vi "add plugin to configuration.vi"(8 "error in (no error)":errorcluster, 9 "plugin info":T1, 10 "id":string, 11 "DSFConfiguration in":refnum<class "DSFConfiguration.lvclass">) -> (0 "error out":errorcluster, 3 "DSFConfiguration out":refnum<class "DSFConfiguration.lvclass">)   [LabVIEW 2017, in "DSFConfiguration.lvclass"]
uses:
  DSFConfiguration.lvclass
  Controls/dsf plugin.ctl
  Controls/dsf timing.ctl
  DSFConfiguration.lvclass/DSFConfiguration.ctl
  DSFPlugin/DSFPlugin.lvclass
  C:/github/data-sharing-framework/Source/Configuration API/Classes/IDable/IDable.lvclass
  IDable/IDable.lvclass/IDable.ctl
  ID API/ID API.lvclass
  IDable/IDable.lvclass
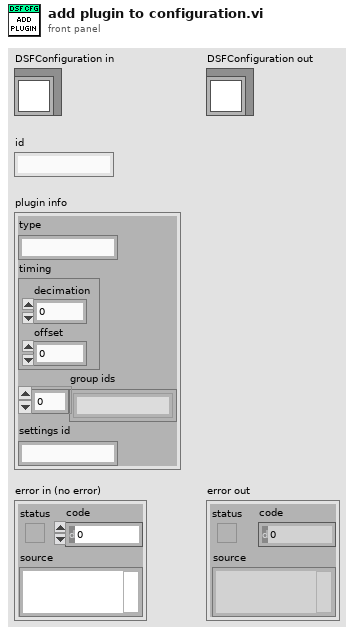
[diagram p1: front panel]
types:
  T1 = typedef "dsf plugin.ctl" = cluster{"type":string, "timing":T2, "group ids":string[], "settings id":string}
  T2 = typedef "dsf timing.ctl" = cluster{"decimation":i32, "offset":i32}
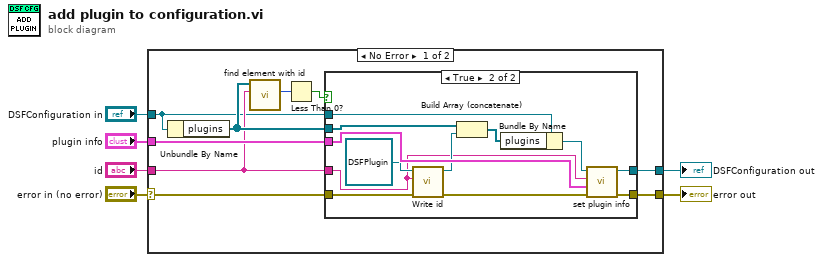
[diagram p0: block diagram]
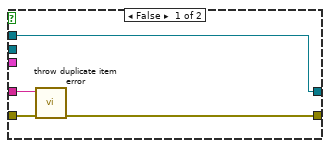
[diagram p2: hidden frame]
diagram:
  n1 = case shown="No Error" "error in (no error)" {
    selector: "error in (no error)" -> [w11 w33]
    tunnel: [w12 w33] -> w1
    tunnel: "DSFConfiguration in" -> [w7 w32]
    tunnel: "id" -> [w9 _]
    tunnel: "plugin info" -> [w10 _]
    tunnel: [w8 w32] -> w2
    frame No Error {
      n2 = Unbundle By Name(w7) -> ("plugins"=w13:refnum<class "DSFPlugin.lvclass">[])
      n3 = call "find element with id.vi"("id"=w9, "IDable Array in"=w13) -> ("index"=w15:i32)  [unwired: 8 in, 1 out]
      n4 = Less Than 0?(x=w15) -> (x < 0?=w14:bool)
      n5 = case shown="True" w14 {
        tunnel: w13 -> [_ w31]
        tunnel: [w19 w26] -> w12
        tunnel: w11 -> [w16 w30]
        tunnel: w10 -> [_ w24]
        tunnel: w9 -> [w17 w20]
        tunnel: w7 -> [w18 w29]
        tunnel: [w18 w25] -> w8
        frame False {
          n6 = call "throw duplicate item error.vi"("error in (no error)"=w16, "id"=w17) -> ("error out"=w19:errorcluster)  [unwired: 9 in]
        }
        frame True {
          n7 = call "Write id.vi"("error in (no error)"=w30, "id"=w20, "IDable in"=refnum<class "DSFPlugin.lvclass"> refnum ("DSFPlugin.lvclass")) -> ("error out"=w23:errorcluster, "IDable out"=w21:refnum<class "DSFPlugin.lvclass">)  [unwired: 7 in]
          n8 = Build Array (concatenate)(w31, w21) -> (w28:refnum<class "DSFPlugin.lvclass">[])
          n9 = Bundle By Name(cluster=w29, "plugins"=w28) -> (w27:refnum<class "DSFConfiguration.lvclass">)
          n10 = call "set plugin info.vi"("error in (no error)"=w23, "plugin info"=w24, "id"=w20, "DSFConfiguration in"=w27) -> ("error out"=w26:errorcluster, "DSFConfiguration out"=w25:refnum<class "DSFConfiguration.lvclass">)  [unwired: 6 in]
        }
      }
    }
    frame Error {
    }
  }
  "error out" <- w1
  "DSFConfiguration out" <- w2
